vi "subsystemControlLoop.vi"() -> ()   [LabVIEW 2020]
uses:
  <vilib>/Simulation/Scripting/Companion Diagram/SimConfigNode/SimParams.ctl
  <vilib>/Simulation/Scripting/Companion Diagram/SimConfigNode/_simSolvers.ctl
  <vilib>/Simulation/Implementation/Shared/SIMSCR Execution Mode.ctl
  <vilib>/Platform/TimedLoop/XDataNode/timing_clust.ctl
  <vilib>/Platform/TimedLoop/XDataNode/nitl_modes.ctl
  <vilib>/Platform/TimedLoop/XDataNode/wakeup.ctl
  <vilib>/Simulation/Param Hierarchy/Typedefs/SIMPH Param Control Actions.ctl
  <vilib>/Simulation/Implementation/Shared/NILVSim_ParamChanged.vi
  <vilib>/Simulation/Implementation/Shared/NILVSim_FinishedLate.vi
  <vilib>/Simulation/Implementation/Shared/NILVSIM_BeginStep.vi
  <vilib>/Simulation/SignalDisplay/Implementation/NILVSim Time Waveform.llb/SIM Time Waveform (vector).vi
  <vilib>/Simulation/Implementation/Shared/NILVSim_Manager.vi
  <vilib>/Utility/error.llb/Clear Errors.vi
  <vilib>/Simulation/Implementation/Shared/NILVSim_FinalizeModel.vi
  <vilib>/Simulation/Implementation/Shared/SIM Unbundle Sim Info.vi
  <vilib>/Simulation/Implementation/Shared/SIMSH Read Queue.vi
  <vilib>/Simulation/Implementation/Shared/NILVSim_Initialize.vi
  <vilib>/Simulation/Utility/Implementation/NILVSim Get Time and IsAcceptedStep.vi
  <vilib>/Simulation/Implementation/Shared/NILVSim_GetModelError.vi
  <vilib>/Simulation/Implementation/Shared/SIM Bundle Sim Info.vi
  <vilib>/Simulation/Scripting/Companion Diagram/SimConfigNode/SimDog.xnode
  Subsystem 2.vi
  <vilib>/Platform/TimedLoop/XDataNode/XDataNode.xnode
  <vilib>/Simulation/Implementation/XNodeFramework/SimXNode/SimX.xnode
  <vilib>/Platform/TimedLoop/XDataNode/XDNodeRunTimeDep.lvlib
  <vilib>/Simulation/Implementation/Shared/NI_SIM_Implementation.lvlib
panel:
  in  "Page Indicator":T1(tab)
  in  "Stop Loop":bool
  in  "Power Percentage":dbl(slide) scale=0.0..100.0
  in  "Inlet Temperature":dbl(knob) scale=20.0..90.0
  out "Inlet and Outlet Temp (0 - 100C)":waveform(dbl)[](graph)
  in  "Select Transfer Function Type":T2(ring)
  out "Inlet and Outlet Temp (250-1000C)":waveform(dbl)[](graph)
  out "Process Power Meter":dbl(knob) scale=0.0..30000.0
  out "Process Output\nPower  (W)":dbl
  out "Temperature Out":dbl
  out "Process Output\nPower":dbl(knob) scale=0.0..5000.0
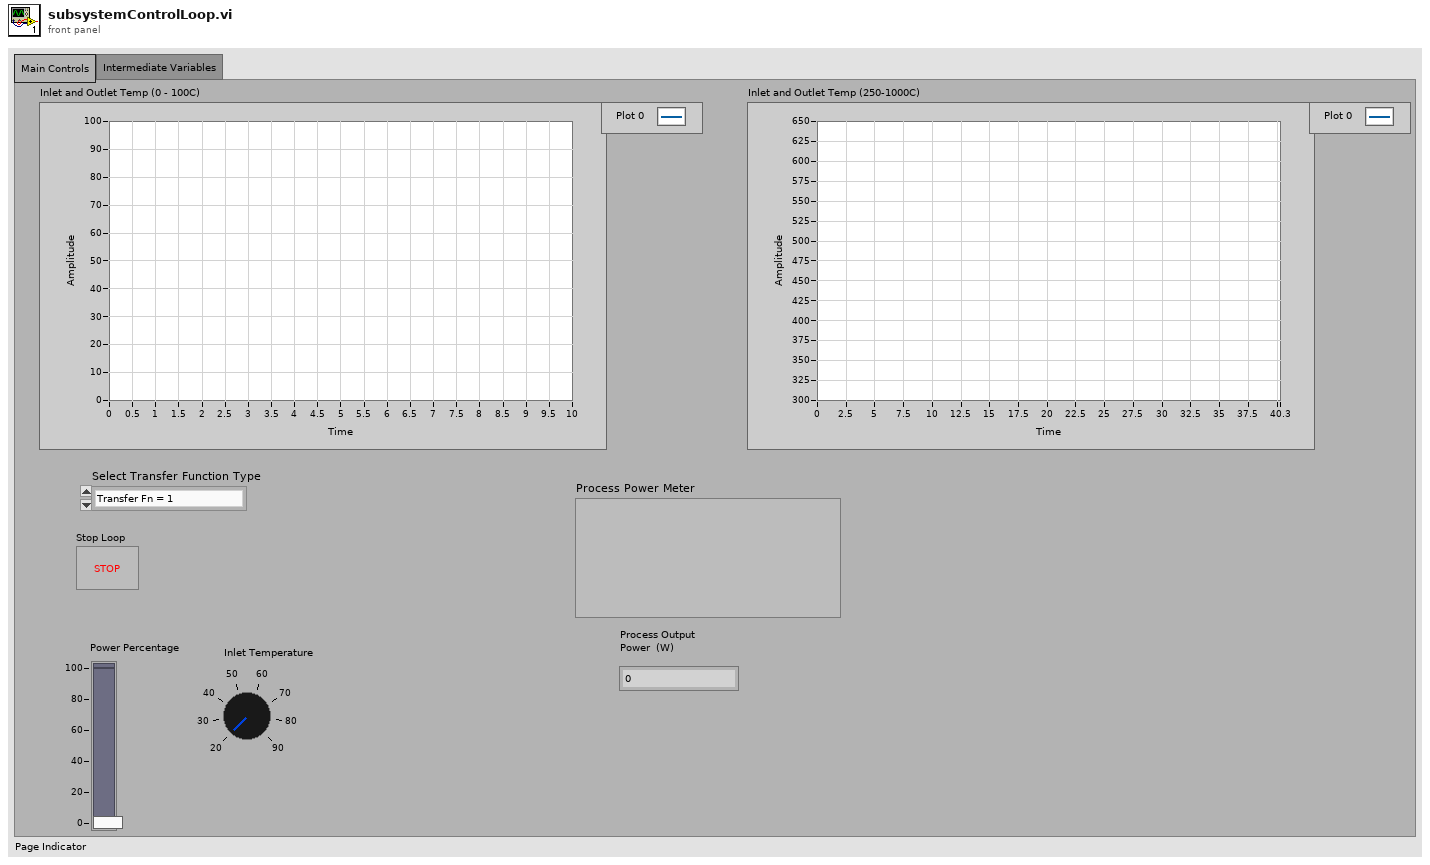
[diagram p1: front panel]
types:
  T1 = enum32{"Main Controls", "Intermediate Variables"}
  T2 = enum16{"Transfer Fn = 1", "First Order with Delay", "Second  Order Transfer Fn", "MISO Trf fn example", "Heater", "Haber Process Mockup"}
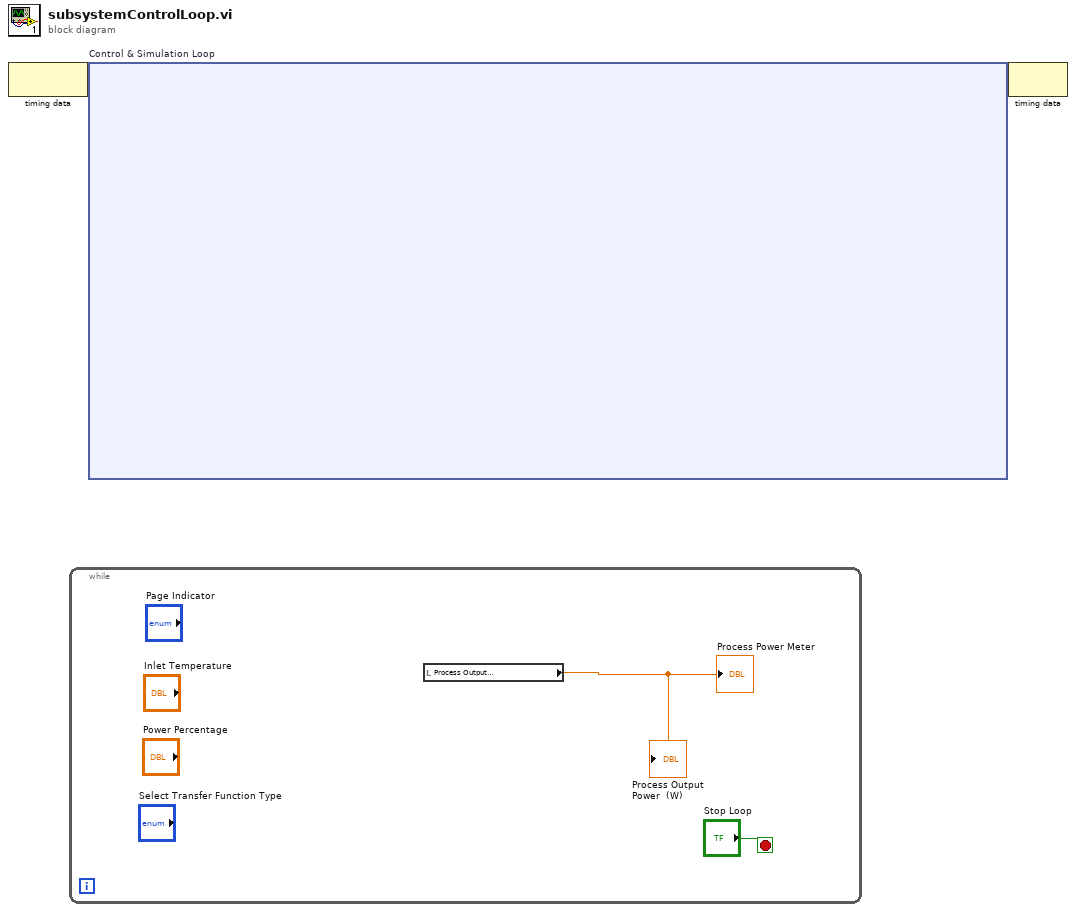
[diagram p0: block diagram]
diagram:
  n1 = node-c288() -> (w2:variant)  [unwired: 1 in]
  n2 = while {
    stop <- "Stop Loop" stop-if-true
    n3 = local read "Process Output\nPower"() -> (→"Process Power Meter" →"Process Output\nPower  (W)":dbl)
  }
  n4 = node-c254 "Control & Simulation Loop"(w2) -> (w1:variant)
  n5 = node-c288(w1) -> ()  [unwired: 1 out]
